vi "Cubic Profile Lookup Setpoints.vi"(9 "Distance":dbl, 11 "Current Time":dbl) -> (1 "Acceleration":dbl, 3 "Velocity":dbl, 4 "Complete?":bool)   [LabVIEW 2015]
uses:
  <vilib>/Rock Robotics/Network Tables/NT Read Number.vi
panel:
  out "Total Time":dbl
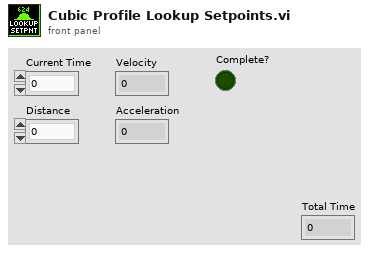
[diagram p1: front panel]
types:
  T1 = typedef "Cubic Motion State.ctl" = enum16{"Stage 1", "Stage 2", "Stage 3", "Stage 4", "Stage 5", "Stage 6", "Stage 7", "Complete"}
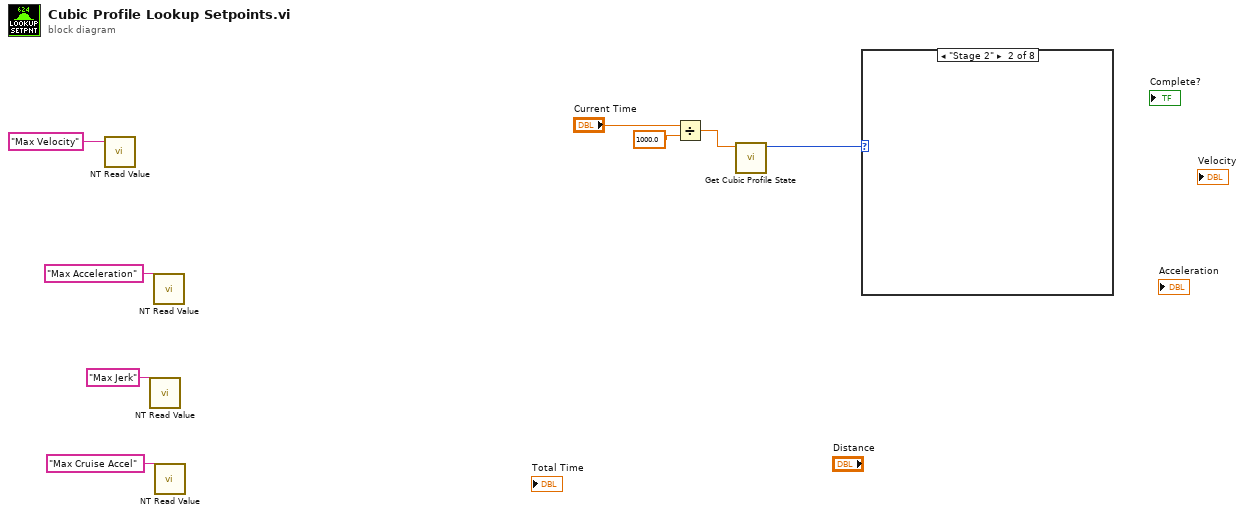
[diagram p0: block diagram]
diagram:
  n1 = call-poly <vilib>:"NT Read Value.vi"("Name"="Max Velocity") -> ()  [unwired: 9 in, 2 out]
  n2 = call-poly <vilib>:"NT Read Value.vi"("Name"="Max Jerk") -> ()  [unwired: 9 in, 2 out]
  n3 = call-poly <vilib>:"NT Read Value.vi"("Name"="Max Acceleration") -> ()  [unwired: 9 in, 2 out]
  n4 = call-poly <vilib>:"NT Read Value.vi"("Name"="Max Cruise Accel") -> ()  [unwired: 9 in, 2 out]
  n5 = Divide(x="Current Time", y=sgl 1000.0) -> (x/y=w6:dbl)
  n6 = call "Get Cubic Profile State.vi"("Current Time"=w6) -> ("Current Stage"=w5:T1)  [unwired: 10 in]
  n7 = case shown="\"Stage 2\"" w5 {
    frame "Stage 1", Default {
    }
    frame "Stage 2" {
    }
    frame "Stage 3" {
    }
    frame "Stage 4" {
    }
    frame "Stage 5" {
    }
    frame "Stage 6" {
    }
    frame "Stage 7" {
    }
    frame "Complete" {
    }
  }
